vi "Discrete Transfer Function.vi"   [LabVIEW 2020, in "NI_AdvCtrl_discrete linear.lvlib"]
doc: "LabVIEW no longer supports this VI. You can obtain similar functionality by installing the LabVIEW Simulation Module.\n\nCalculates the new output point, where the transfer function and the input point are given. The transfer function is described by two polynomials, numerator and denominator."
uses:
  <vilib>/addons/control/advanced/NI_AdvCtrl_discrete linear.lvlib
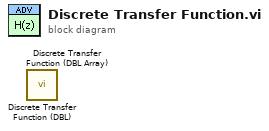
[diagram p0: block diagram]
diagram:
  n1 = call <vilib>:"Discrete Transfer Function (DBL).vi"() -> ()  [unwired: 5 in, 1 out]
  n2 = call <vilib>:"Discrete Transfer Function (DBL Array).vi"() -> ()  [unwired: 5 in, 1 out]
